vi "int_string.vi"(11 "Numeric":dbl) -> (3 "%06.6e string out":string)   [LabVIEW 2016]
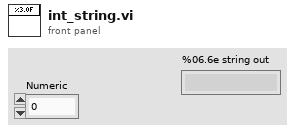
[diagram p1: front panel]
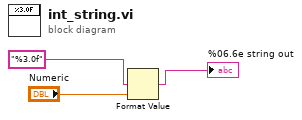
[diagram p0: block diagram]
diagram:
  n1 = Format Value(format string="%3.0f", value (0)="Numeric") -> (output string=→"%06.6e string out":string)  [unwired: 1 in]
